vi "LoadPatientDateInfo_File.vi"(8 "error in (no error)":errorcluster, 11 "DataPatientDatePath":path) -> (0 "error out":errorcluster, 2 "date_specific_info":T1, 3 "path":path)   [LabVIEW 2013, in "main.lvlib"]
uses:
  main.lvlib
  Controls/date_specific_info.ctl
  Controls/Enum User Events.ctl
  Globals/DataPathGlobalVariable.vi
  <userlib>/_OpenG.lib/file/file.llb/File Exists - Scalar__ogtk.vi
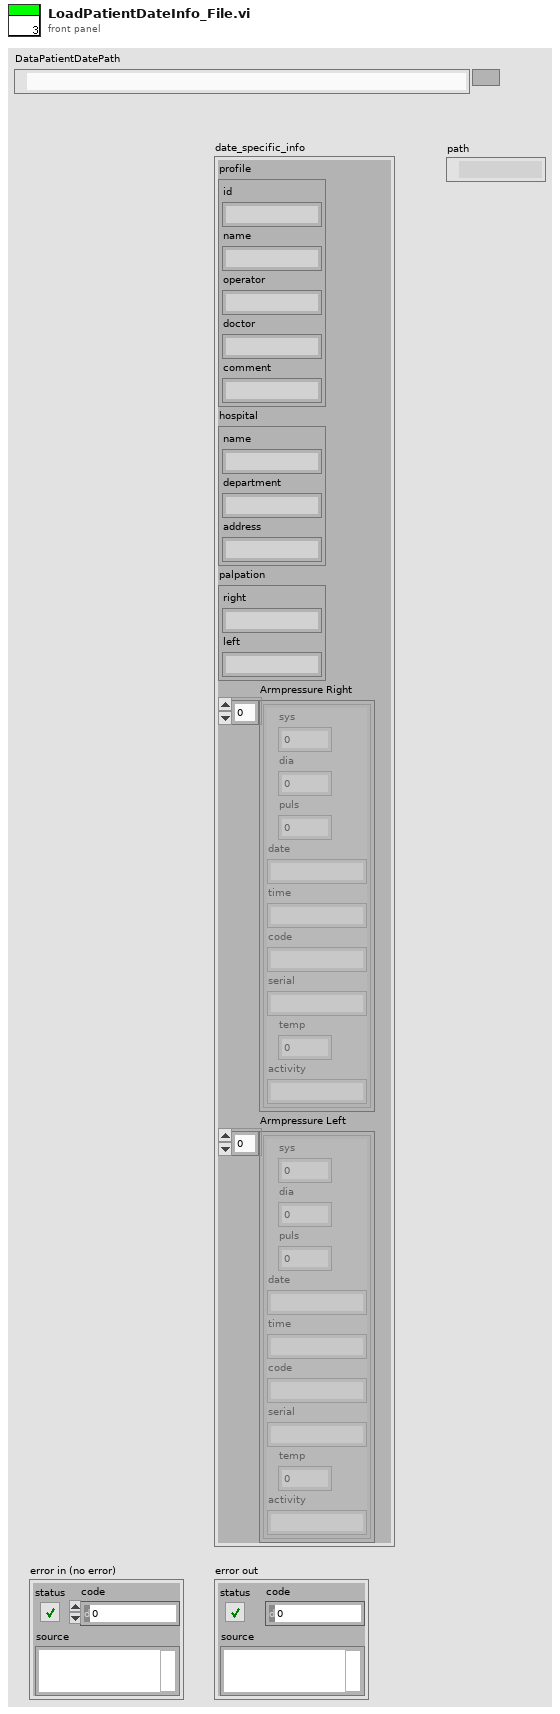
[diagram p1: front panel]
types:
  T1 = typedef "main.lvlib/date_specific_info.ctl" = cluster{"profile":cluster{"id":string, "name":string, "operator":string, "doctor":string, "comment":string}, "hospital":cluster{"name":string, "department":string, "address":string}, "palpation":cluster{"right":string, "left":string}, "Armpressure Right":cluster{"sys":dbl, "dia":dbl, "puls":dbl, "date":string, "time":string, "code":string, "serial":string, "temp":dbl, "activity":string}[], "Armpressure Left":cluster{"sys":dbl, "dia":dbl, "puls":dbl, "date":string, "time":string, "code":string, "serial":string, "temp":dbl, "activity":string}[]}
  T2 = enum16{"open", "replace", "create", "open or create", "replace or create", "replace or create with confirmation"}
  T3 = typedef "main.lvlib/Enum User Events.ctl" = enum16{"User Event", "Init"}
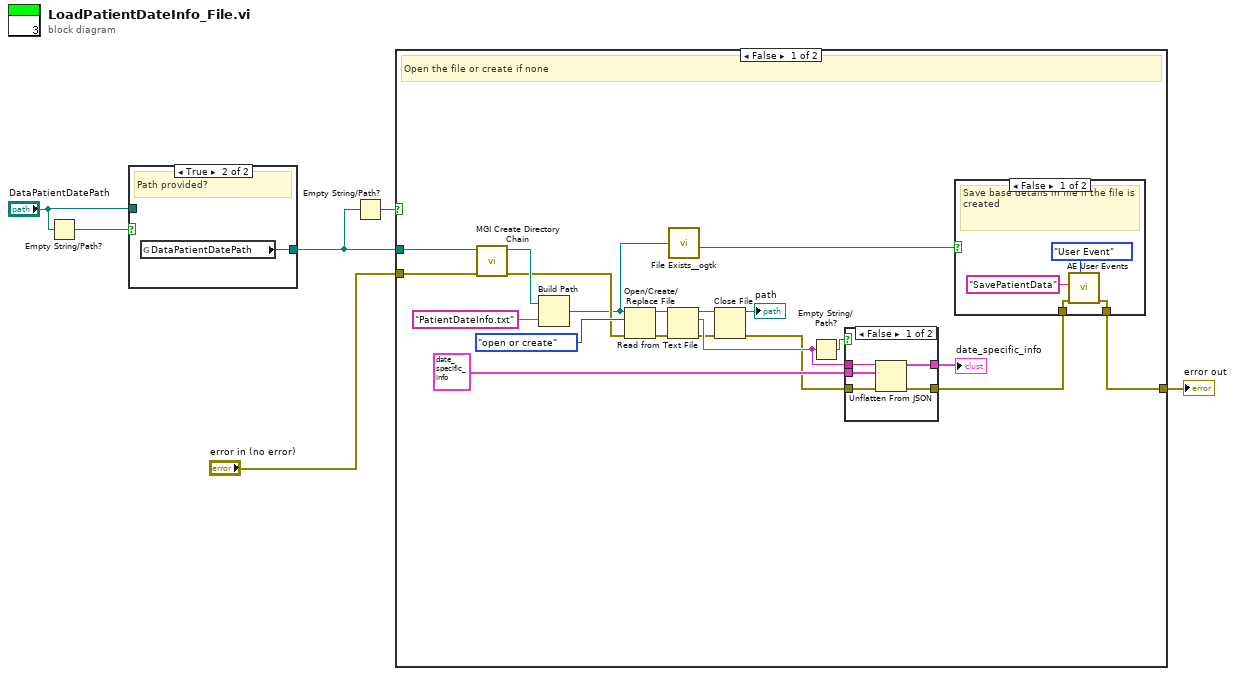
[diagram p0: block diagram]
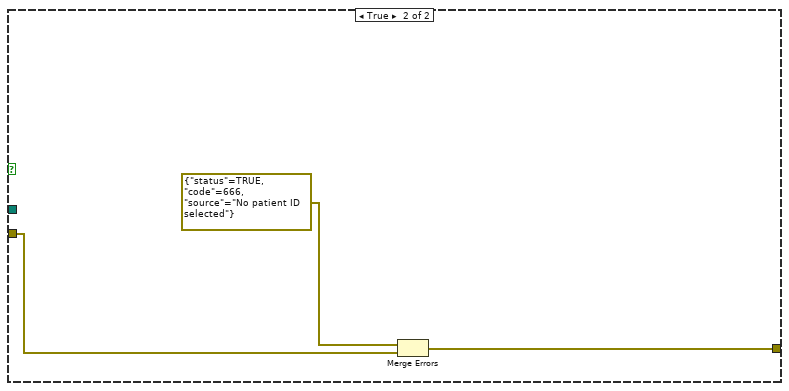
[diagram p5: hidden frame]
diagram:
  n1 = Empty String/Path?(string/path="DataPatientDatePath") -> (empty?=w3:bool)
  n2 = case shown="True" w3 {
    tunnel: [w7 w8] -> w2
    tunnel: "DataPatientDatePath" -> [w7 _]
    frame False {
    }
    frame True {
      # "Path provided?"
      n3 = global read "DataPathGlobalVariable.vi" "DataPatientDatePath"() -> (w8:path)
    }
  }
  n4 = Empty String/Path?(string/path=w2) -> (empty?=w4:bool)
  n5 = case shown="False" w4 {
    tunnel: [w10 w43] -> w6
    tunnel: w2 -> [w15 _]
    tunnel: "error in (no error)" -> [w13 w41]
    frame False {
      # "Open the file or create if none"
      n6 = call <userlib>:"MGI Create Directory Chain.vi"("Error In"=w13, "Path"=w15) -> ("Error Out"=w14:errorcluster, "Duplicate Path"=w16:path)  [unwired: 8 in]
      n7 = Build Path(base path=w16, name or relative path="PatientDateInfo.txt") -> (appended path=w12:path)
      n8 = Open/Create/Replace File(file path (use dialog)=w12, error in=w14, operation (0:open)=T2."open or create") -> (refnum out=w24:refnum<file>, error out=w23:errorcluster)  [unwired: 3 in, 1 out]
      n9 = Read from Text File(file (use dialog)=w24, error in=w23) -> (refnum out=w20:refnum<file>, text=w26:string, error out=w19:errorcluster)  [unwired: 2 in, 1 out]
      n10 = call-poly <userlib>:"File Exists__ogtk.vi"("file path"=w12) -> ("exists"=w9:bool)  [unwired: 6 in, 1 out]
      n11 = Close File(refnum=w20, error in=w19) -> (path=→"path":path, error out=w18:errorcluster)
      n12 = Empty String/Path?(string/path=w26) -> (empty?=w27:bool)
      n13 = case shown="False" w27 {
        tunnel: T1 {"profile"={"id"="", "name"="", "operator"="", "doctor"="", "comment"=""}, "hospital"={"name"="", "department"="", "address"=""}, "palpation"={"right"="", "left"=""}, "Armpressure Right"=[], "Armpressure Left"=[]} ("date_specific_info") -> [w38 w40]
        tunnel: w26 -> [w37 _]
        tunnel: w18 -> [w36 w39]
        tunnel: [w35 w40] -> w28
        tunnel: [w34 w39] -> w11
        frame False {
          n14 = Unflatten From JSON(JSON string=w37, type and defaults=w38, error in (no error)=w36) -> (value=w35:T1, error out=w34:errorcluster)  [unwired: 4 in]
        }
        frame True {
        }
      }
      "date_specific_info" <- w28
      n15 = case shown="False" w9 {
        tunnel: w11 -> [w32 w33]
        tunnel: [w31 w33] -> w10
        frame False {
          # "Save base details in file if the file is created"
          n16 = call "AE User Events.vi"("Action"=Enum_User_Events."User Event", "error in (no error)"=w32, "User Event"="SavePatientData") -> ("error out"=w31:errorcluster)  [unwired: 7 in, 1 out]
        }
        frame True {
        }
      }
    }
    frame True {
      n17 = Merge Errors(errorcluster {"status"=TRUE, "code"=666, "source"="No patient ID selected"} ("error in (no error)"), w41) -> (w43:errorcluster)
    }
  }
  "error out" <- w6
